vi "Set Display Basetime.vi"(8 "error in (no error)":errorcluster, 10 "Basetime":T1(ring), 11 "VISA resource name":refnum<visa-resource-name>) -> (0 "error out":errorcluster, 3 "VISA resource name out":refnum<visa-resource-name>)   [LabVIEW 2017, in "Sefram DAS220.lvlib"]
doc: "Change the basetime for F(t) graphic from 100 millisec/div to 20 minutes/div."
uses:
  <instrlib>/Sefram DAS220/Sefram DAS220.lvlib
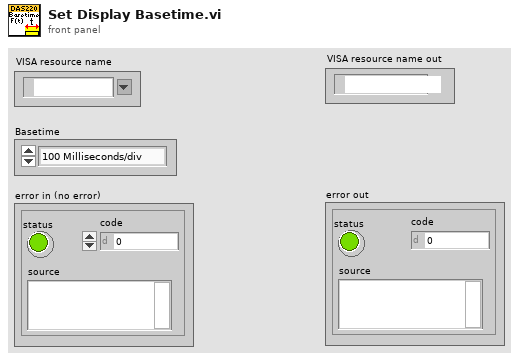
[diagram p1: front panel]
types:
  T1 = enum16{"100 Milliseconds/div", "200 Milliseconds/div", "500 Milliseconds/div", "1 Second/div", "2 Seconds/div", "5 Seconds/div", "10 Seconds/div", "20 Seconds/div", "1 Minute/div", "2 Minutes/div", "5 Minutes/div", "10 Minutes/div", "20 Minutes/div"}
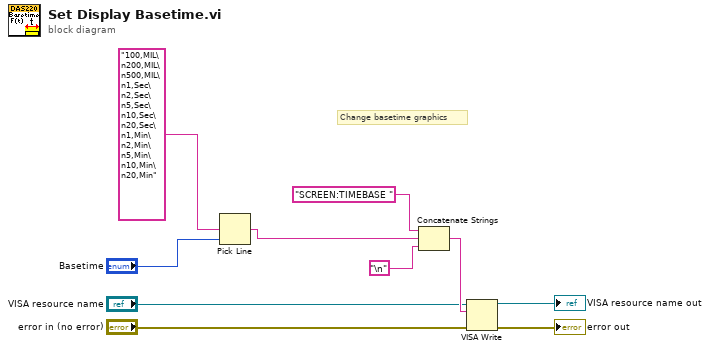
[diagram p0: block diagram]
diagram:
  # "Change basetime graphics"
  n1 = Pick Line(multi-line string="100,MIL\n200,MIL\n500,MIL\n1,Sec\n2,Sec\n5,Sec\n10,Sec\n20,Sec\n1,Min\n2,Min\n5,Min\n10,Min\n20,Min", line index="Basetime") -> (output string=w7:string)  [unwired: 1 in]
  n2 = Concatenate Strings("SCREEN:TIMEBASE " ("string"), w7, "\n") -> (w10:string)
  n3 = VISA Write(VISA resource name="VISA resource name", write buffer=w10, error in (no error)="error in (no error)") -> (VISA resource name out=→"VISA resource name out":refnum<visa-resource-name>, error out=→"error out":errorcluster)  [unwired: 1 out]
